vi "nanocal -- nuclear schottky fit V5.vi"() -> ()   [LabVIEW 2020] (continued)
  n20 = Bundle By Name(cluster=T15 {"left"=0.0, "right "=0.0, "center"=0.0, "window"=0.0, "cursors"=[], "relative"=0, "absolute"=0, "fixed vertical offset"=0.0, "vertical offset"=0.0, "skew"=0.0, "default window frac"=0.0, "kind"=enum."symmetric", "skew.left"=0.0, "skew.right"=0.0, "Plot ref"=refnum, "wing order"=enum."forw"} ("cursor bracket: All, data window"), "Plot ref"=w25, "cursors"=i32[] [0, 1, 2], "fixed vertical offset"=0.0, "default window frac"=0.3 ("fixed vertical offset"), "kind"=enum16{"symmetric", "skewed", "fancy"}."symmetric") -> (w28:T15)
  n21 = local write "factors"(cluster{"scaling":dbl, "what":T1}[] [{"scaling"=1.0, "what"=enum."ζ"}, {"scaling"=1.0, "what"=enum."τ1"}, {"scaling"=1.0, "what"=enum."τS"}, {"scaling"=1.0, "what"=enum."τN"}, {"scaling"=1.0, "what"=enum."τC"}, {"scaling"=1.0, "what"=enum."κ0"}]) -> ()
  n22 = control-ref of="cursor window"() -> (w24:refnum<vi>)
  n23 = call "cursor window logic V3.vi"("cursor window action"=cursor_window_action."init", "cursor window in"=w24, "cursor window init"=w28) -> ()  [unwired: 7 in, 2 out]
  n24 = Create User Event(user event datatype=w33) -> (user event=w14:refnum<user-event>)  [unwired: 1 in, 1 out]
  n25 = Bundle(w13, w13) -> (w12:cluster{dbl[], dbl[]})  [unwired: 1 in]
  n26 = Initialize Array(w12, 5 ("dimension size")) -> (→"Plot: goodness vs parameter":cluster{dbl[], dbl[]}[])
  n27 = control-ref of="Plot: sweep window"() -> (w20:refnum<vi>)
  n28 = register-events(w14) -> (reference out=w34:refnum<event-registration>)  [unwired: 2 in, 1 out]
  n29 = Create User Event(user event datatype=w35) -> (user event=w23:refnum<user-event>)  [unwired: 1 in, 1 out]
  n30 = register-events(w23) -> (reference out=w36:refnum<event-registration>)  [unwired: 2 in, 1 out]
  n31 = local write "newton pause"(w16) -> ()
  n32 = control-ref of="Plot:  colors"() -> (w17:refnum<vi>)
  n33 = local write "default selector"(w5) -> ()
  n34 = call "replace cursor - plot ref - V2.vi"("Plot ref in"=w20, "new X"=w19, "new  Y"=w19, "cursor index"=2, "cursor action"=cursor_action."write") -> ()  [unwired: 11 in, 4 out]
  n35 = local write "parameter"(w4) -> ()
  n36 = while "actions" {
    tunnel: w36 -> [w96]
    tunnel: w23 -> [w95]
    tunnel: w14 -> [w93]
    tunnel: w4 -> [w92]
    tunnel: w5 -> [w91]
    stop <- w94 stop-if-true
    n37 = event shown="[0] <action>: User Event" {
      selector: w96 -> [_]
      dyn-events: _ -> [_]
      timeout: _ -> [_]
      tunnel: w95 -> [w101]
      tunnel: [w100] -> w94
      tunnel: w93 -> [w99]
      tunnel: w92 -> [w98]
      tunnel: w91 -> [w97]
      event User Event {
        n38 = event-data() -> ("action"=w102:string)  [unwired: 1 in]
        n39 = case shown="\"action: replot circles\"" w102 {
          tunnel: w101 -> [w114 _ _ w322 w424 w442 w467 _ _ w660 _ w786 _ _ w937 _ w1008 w1100 _ w1157 _ _]
          tunnel: [_ _ _ _ _ _ _ _ _ _ _ _ _ _ _ _ _ _ TRUE _ _ _] -> w100
          tunnel: w99 -> [_ _ _ _ _ _ _ _ _ _ _ _ _ _ _ _ _ _ _ _ _ _]
          tunnel: w98 -> [w105 w174 w202 _ _ _ _ w594 _ _ _ _ _ w833 _ _ w1004 _ _ _ _ _]
          tunnel: w97 -> [_ _ _ _ _ _ _ _ _ _ _ _ _ _ _ _ _ _ _ _ _ _]
          frame "action: new sweep" {
            w117 = T1[] [enum."m1", enum."m2", enum."m3"] items=["ζ", "τ1", "τS", "τN", "τC", "κ0", "m1", "m2", "m3", "T (K)", "B (T)", "θ (deg)", "side (S|R)", "set of (B|T)", "Re(offset)", "Im(offset)"]
            w123 = T1[] [enum."T (K)", enum."B (T)", enum."θ (deg)"] items=["ζ", "τ1", "τS", "τN", "τC", "κ0", "m1", "m2", "m3", "T (K)", "B (T)", "θ (deg)", "side (S|R)", "set of (B|T)", "Re(offset)", "Im(offset)"]
            n40 = local read "τN"() -> (w143:dbl)
            n41 = local read "τC"() -> (w142:dbl)
            n42 = local read "T1"() -> (w145:dbl)
            n43 = local read "κ0"() -> (w141:dbl)
            n44 = local read "τS"() -> (w144:dbl)
            n45 = local read "ζ"() -> (w146:dbl)
            n46 = Generate User Event(user event=w114, event data cluster="action: reset colors" ("event data")) -> ()  [unwired: 2 in, 2 out]
            n47 = Build Array (concatenate)(w105, w117) -> (w116:T1[])
            n48 = Build Array(w146, w145, w144, w143, w142, w141) -> (w129:dbl[])
            n49 = local read "newton parameters"() -> (w110:T2)
            n50 = for {
              shift-right: [w158] -> w106
              shift-left: map{T1, dbl} {} ("Map IN") -> [w159]
              tunnel: w116 -> [w156] mode=indexing
              tunnel: w129 -> [w157] mode=indexing
              tunnel: [w156] -> w118 mode=indexing
              n51 = Insert Into Map(map in=w159, key=w156, value=w157) -> (map out=w158:map{T1, dbl})  [unwired: 2 out]
            }
            n52 = local read "θ (deg)"() -> (w125:dbl)
            n53 = local read "B (T)"() -> (w126:dbl)
            n54 = local read "T (K)"() -> (w127:dbl)
            n55 = call "nanocal -- publish -- freq scan V2.vi"("publisher action"=publisher_action."get") -> ("z out (V)"=w112:cdb[], "data"=w103:T30)  [unwired: 7 in, 2 out]
            n56 = Build Array(w127, w126, w125) -> (w122:dbl[])
            n57 = call "3-lorentzian-heat-response -- V4.vi"("action"=3-lorentzian-heat-response_action."calc m1m2m3", "Map IN"=w106) -> ("Map OUT"=w124:map{T1, dbl})  [unwired: 7 in, 2 out]
            n58 = for {
              shift-right: [w154] -> w121
              shift-left: w124 -> [w155]
              tunnel: w123 -> [w153] mode=indexing
              tunnel: w122 -> [w152] mode=indexing
              n59 = Insert Into Map(map in=w155, key=w153, value=w152) -> (map out=w154:map{T1, dbl})  [unwired: 2 out]
            }
            n60 = control-ref of="Plot: sweep window"() -> (w140:refnum<vi>)
            n61 = call "nanocal -- gradient descent.vi"("data"=w103, "action"=nanocal_--_gradient_descent_--_action."peek", "newton pars"=w110, "parameter keys IN"=w105, "parameter Map IN"=w106) -> ("logarithmic derivatives OUT"=→"logarithmic derivatives":dbl[], "R(ω) out"=w108:cdb[], "goodness OUT"=→"goodness":dbl)  [unwired: 2 in, 2 out]
            n62 = local read "cursor x selector"() -> (w150:map{T1, dbl})
            n63 = local read "X selector"() -> (w149:T1)
            n64 = local read "cursor index map"() -> (w130:map{T1, i32})
            n65 = Complex To Re/Im(x + iy=w112) -> (x=w139:dbl[], y=w138:dbl[])
            n66 = local read "T (K)"() -> (w148:dbl)
            n67 = call "string parse mathematica assosiated array.vi"("action"=mathematica_string_map_action."create string" ("derivative"), "map IN"=w121) -> ("String OUT"=w119:string)  [unwired: 8 in, 1 out]
            n68 = control-ref of="Plot:  colors"() -> (w151:refnum<vi>)
            n69 = local write "String"(w119) -> ()
            n70 = call "replace plot - plot ref - V2.vi"("Plot ref in"=w140, "Array X IN"=w139, "Array Y IN"=w138, "plot index"=enum16{"data R(ω)", "fit R(ω)"}."data R(ω)" ("Plost: sweep window"), "cursor action"=cursor_action."write") -> ("Plot ref out"=w137:refnum<vi>)  [unwired: 11 in, 3 out]
            n71 = Complex To Re/Im(x + iy=w108) -> (x=w135:dbl[], y=w134:dbl[])
            n72 = Look In Map(map=w150, key=w149, default value=w148) -> (value=w147:dbl)  [unwired: 1 out]
            n73 = for {
              tunnel: w147 -> [w167]
              tunnel: w151 -> [w166]
              tunnel: w118 -> [w162] mode=indexing
              tunnel: w130 -> [w164]
              shift-right: [w161] -> _
              shift-left: w124 -> [w161]
              n74 = Look In Map(map=w161, key=w162) -> (value=w160:dbl)  [unwired: 1 in, 1 out]
              n75 = Look In Map(map=w164, key=w162) -> (value=w163:i32)  [unwired: 1 in, 1 out]
              n76 = call "replace cursor - plot ref - V2.vi"("Plot ref in"=w166, "new X"=w167, "new  Y"=w160, "cursor index"=w163, "cursor action"=cursor_action."write") -> ()  [unwired: 11 in, 4 out]
            }
            n77 = call "replace plot - plot ref - V2.vi"("Plot ref in"=w137, "Array X IN"=w135, "Array Y IN"=w134, "plot index"=enum16{"data R(ω)", "fit R(ω)"}."fit R(ω)" ("Plost: sweep window"), "cursor action"=cursor_action."write") -> ()  [unwired: 11 in, 4 out]
          }
          frame "action: replot circles" {
            n78 = local read "τN"() -> (w193:dbl)
            n79 = local read "τC"() -> (w192:dbl)
            n80 = local read "T1"() -> (w195:dbl)
            n81 = local read "κ0"() -> (w191:dbl)
            n82 = local read "τS"() -> (w194:dbl)
            n83 = local read "ζ"() -> (w196:dbl)
            n84 = local read "newton parameters"() -> (w177:T2)
            n85 = Build Array(w196, w195, w194, w193, w192, w191) -> (w171:dbl[])
            n86 = call "nanocal -- publish -- freq scan V2.vi"("publisher action"=publisher_action."get") -> ("z out (V)"=w176:cdb[], "data"=w172:T30)  [unwired: 7 in, 2 out]
            n87 = for {
              shift-right: [w199] -> w173
              shift-left: map{T1, dbl} {} ("Map IN") -> [w200]
              tunnel: w174 -> [w198] mode=indexing
              tunnel: w171 -> [w197] mode=indexing
              n88 = Insert Into Map(map in=w200, key=w198, value=w197) -> (map out=w199:map{T1, dbl})  [unwired: 2 out]
            }
            n89 = call "nanocal -- gradient descent.vi"("data"=w172, "action"=nanocal_--_gradient_descent_--_action."peek", "newton pars"=w177, "parameter keys IN"=w174, "parameter Map IN"=w173) -> ("logarithmic derivatives OUT"=w169:dbl[], "R(ω) out"=w175:cdb[], "goodness OUT"=w170:dbl)  [unwired: 2 in, 2 out]
            n90 = control-ref of="Plot: sweep window"() -> (w188:refnum<vi>)
            n91 = local write "logarithmic derivatives"(w169) -> ()
            n92 = local write "goodness"(w170) -> ()
            n93 = Complex To Re/Im(x + iy=w176) -> (x=w186:dbl[], y=w185:dbl[])
            n94 = call "replace plot - plot ref - V2.vi"("Plot ref in"=w188, "Array X IN"=w186, "Array Y IN"=w185, "plot index"=enum16{"data R(ω)", "fit R(ω)"}."data R(ω)" ("Plost: sweep window"), "cursor action"=cursor_action."write") -> ("Plot ref out"=w187:refnum<vi>)  [unwired: 11 in, 3 out]
            n95 = Complex To Re/Im(x + iy=w175) -> (x=w184:dbl[], y=w183:dbl[])
            n96 = Absolute Value(x=w169) -> (abs(x)=w168:dbl[])
            n97 = local write "log(|dlogG/dlogα|)"(w168) -> ()
            n98 = call "replace plot - plot ref - V2.vi"("Plot ref in"=w187, "Array X IN"=w184, "Array Y IN"=w183, "plot index"=enum16{"data R(ω)", "fit R(ω)"}."fit R(ω)" ("Plost: sweep window"), "cursor action"=cursor_action."write") -> ()  [unwired: 11 in, 4 out]
          }
          frame "action: plot landscape" {
            w214 = array_action."generate log range" ("action")
            n99 = property on="range one" class="Slide (strict)"() -> ("Scale.Range"=w225:T32)  [unwired: 2 in, 2 out]
            n100 = local read "ζ"() -> (w231:dbl)
            n101 = local read "τS"() -> (w229:dbl)
            n102 = local read "τN"() -> (w228:dbl)
            n103 = local read "τC"() -> (w227:dbl)
            n104 = local read "T1"() -> (w230:dbl)
            n105 = local read "κ0"() -> (w226:dbl)
            n106 = property on="range two" class="Slide (strict)"() -> ("Scale.Range"=w224:T32)  [unwired: 2 in, 2 out]
            n107 = Unbundle By Name(w225) -> ("Maximum"=w217:dbl, "Minimum"=w216:dbl)
            n108 = Unbundle By Name(w224) -> ("Maximum"=w219:dbl, "Minimum"=w218:dbl)
            n109 = Build Array(w231, w230, w229, w228, w227, w226) -> (w213:dbl[])
            n110 = local read "cursor index map"() -> (w208:map{T1, i32})
            n111 = call "array -- generate range -- V5.vi"("action"=w214, "ω points"="# points", "ω from"=w216, "ω to"=w217) -> ("ω out"=w215:dbl[])  [unwired: 7 in]
            n112 = call "array -- generate range -- V5.vi"("action"=w214, "ω points"="# points", "ω from"=w218, "ω to"=w219) -> ("ω out"=w220:dbl[])  [unwired: 7 in]
            n113 = local read "color Map"() -> (w209:map{T1, u32})
            n114 = call "nanocal -- publish -- freq scan V2.vi"("publisher action"=publisher_action."get") -> ("data"=w201:T30)  [unwired: 7 in, 3 out]
            n115 = local read "newton parameters"() -> (w203:T2)
            n116 = for {
              shift-right: [w314] -> w221
              shift-left: map{T1, dbl} {} ("Map IN") -> [w315]
              tunnel: w202 -> [w313] mode=indexing
              tunnel: w213 -> [w312] mode=indexing
              n117 = Insert Into Map(map in=w315, key=w313, value=w312) -> (map out=w314:map{T1, dbl})  [unwired: 2 out]
            }
            n118 = Look In Map(map=w209, key="two") -> (value=w211:u32)  [unwired: 1 in, 1 out]
            n119 = Look In Map(map=w209, key="one") -> (value=w210:u32)  [unwired: 1 in, 1 out]
            n120 = Build Array("one", "two") -> (w207:T1[])
            n121 = property on="range one" class="Slide (strict)"("Fill Color"=w210) -> ()  [unwired: 2 in, 2 out]
            n122 = property on="range two" class="Slide (strict)"("Fill Color"=w211) -> ()  [unwired: 2 in, 2 out]
            n123 = case shown="\"1d plots\", Default" "what" {
              tunnel: w221 -> [w239 w279]
              tunnel: "one" -> [_ w278]
              tunnel: w220 -> [_ w277]
              tunnel: w215 -> [w238 w276]
              tunnel: "two" -> [_ w275]
              tunnel: w209 -> [w237 _]
              tunnel: w208 -> [w236 _]
              tunnel: w207 -> [w233 _]
              tunnel: w201 -> [w234 w270]
              tunnel: w203 -> [w232 w268]
              tunnel: w202 -> [_ w269]
              frame "1d plots", Default {
                n124 = control-ref of="Plot: goodness vs parameter"() -> (w235:refnum<vi>)
                n125 = for {
                  tunnel: w239 -> [w246]
                  tunnel: w238 -> [w255]
                  tunnel: w233 -> [w245] mode=indexing
                  tunnel: w237 -> [w252]
                  tunnel: w236 -> [w251]
                  tunnel: w235 -> [w243]
                  tunnel: w234 -> [w242]
                  tunnel: w233 -> [w241]
                  tunnel: w232 -> [w240]
                  n126 = for {
                    tunnel: w255 -> [w259] mode=indexing
                    tunnel: [w260] -> w257 mode=indexing
                    tunnel: [w259] -> w256 mode=indexing
                    tunnel: w246 -> [w266]
                    tunnel: w245 -> [w267]
                    tunnel: w242 -> [w265]
                    tunnel: w241 -> [w262]
                    tunnel: w240 -> [w261]
                    n127 = Insert Into Map(map in=w266, key=w267, value=w259) -> (map out=w264:map{T1, dbl})  [unwired: 2 out]
                    n128 = call "nanocal -- gradient descent.vi"("data"=w265, "action"=nanocal_--_gradient_descent_--_action."peek", "newton pars"=w261, "parameter keys IN"=w262, "parameter Map IN"=w264) -> ("goodness OUT"=w260:dbl)  [unwired: 2 in, 4 out]
                  }
                  n129 = Look In Map(map=w246, key=w245) -> (value=w244:dbl)  [unwired: 1 in, 1 out]
                  n130 = Look In Map(map=w252, key=w245) -> (value=w247:u32)  [unwired: 1 in, 1 out]
                  n131 = Look In Map(map=w251, key=w245) -> (value=w249:i32)  [unwired: 1 in, 1 out]
                  n132 = call "replace plot - plot ref - V2.vi"("Plot ref in"=w243, "Array X IN"=w256, "Array Y IN"=w257, "plot index"=w249, "cursor action"=cursor_action."write") -> ("Plot ref out"=w254:refnum<vi>)  [unwired: 11 in, 3 out]
                  n133 = call "replace cursor - plot ref - V2.vi"("Plot ref in"=w243, "new X"=w244, "cursor index"=w249, "cursor action"=cursor_action."write", "Color Box"=w247, "cursor state"=cursor_sate."colored") -> ()  [unwired: 10 in, 4 out]
                  n134 = call "replace plot - plot ref - V2.vi"("Plot ref in"=w254, "plot index"=w249, "cursor action"=cursor_action."set plot color", "Color Box"=w247) -> ()  [unwired: 12 in, 4 out]
                }
              }
              frame "2d plots " {
                n135 = for {
                  tunnel: w279 -> [w289]
                  tunnel: w278 -> [w288]
                  tunnel: w277 -> [w287] mode=indexing
                  tunnel: w276 -> [w286]
                  tunnel: w275 -> [w285]
                  shift-right: [w283] -> w272
                  shift-left: "{ " -> [w284]
                  tunnel: w270 -> [w282]
                  tunnel: w269 -> [w281]
                  tunnel: w268 -> [w280]
                  n136 = for {
                    tunnel: w286 -> [w297] mode=indexing
                    tunnel: w287 -> [w296]
                    tunnel: w289 -> [w310]
                    tunnel: w288 -> [w311]
                    tunnel: w285 -> [w309]
                    shift-right: [w306] -> w283
                    shift-left: w284 -> [w307]
                    tunnel: w282 -> [w294]
                    tunnel: w281 -> [w291]
                    tunnel: w280 -> [w290]
                    w300 = " ,     "
                    w305 = i16 12 ("precision (6)")
                    n137 = Insert Into Map(map in=w310, key=w311, value=w297) -> (map out=w308:map{T1, dbl})  [unwired: 2 out]
                    n138 = Number To Fractional String(number=w297, precision (6)=w305) -> (F-format string=w304:string)  [unwired: 2 in]
                    n139 = Number To Fractional String(number=w296, precision (6)=w305) -> (F-format string=w303:string)  [unwired: 2 in]
                    n140 = Insert Into Map(map in=w308, key=w309, value=w296) -> (map out=w295:map{T1, dbl})  [unwired: 2 out]
                    n141 = call "nanocal -- gradient descent.vi"("data"=w294, "action"=nanocal_--_gradient_descent_--_action."peek", "newton pars"=w290, "parameter keys IN"=w291, "parameter Map IN"=w295) -> ("goodness OUT"=w292:dbl)  [unwired: 2 in, 4 out]
                    n142 = Number To Fractional String(number=w292, precision (6)=w305) -> (F-format string=w302:string)  [unwired: 2 in]
                    n143 = Concatenate Strings(w307, "{    ", w304, w300, w303, w300, w302, " } , ", "\r") -> (w306:string)
                  }
                }
                n144 = Concatenate Strings(w272, " }   ") -> (→"2dplots":string)
              }
            }
          }
          frame "action: gradient step" {
            w319 = T1[] [enum."ζ", enum."τ1", enum."τS", enum."τN", enum."τC", enum."κ0"] items=["ζ", "τ1", "τS", "τN", "τC", "κ0", "m1", "m2", "m3", "T (K)", "B (T)", "θ (deg)", "side (S|R)", "set of (B|T)", "Re(offset)", "Im(offset)"]
            w323 = FALSE ("newton pause")
            n145 = local write "newton pause"(w323) -> ()
            n146 = call "nanocal -- publish -- freq scan V2.vi"("publisher action"=publisher_action."get") -> ("data"=w316:T30)  [unwired: 7 in, 3 out]
            n147 = Generate User Event(user event=w322, event data cluster="action: new sweep" ("event data")) -> ()  [unwired: 2 in, 2 out]
            n148 = call "nanocal -- gradient descent.vi"("data"=w316, "action"=nanocal_--_gradient_descent_--_action."init") -> ("goodness OUT"=w320:dbl)  [unwired: 5 in, 4 out]
            n149 = for {
              N: "# steps" -> [_]
              tunnel: [TRUE ("newton pause")] -> w324
              tunnel: w323 -> [_]
              tunnel: w320 -> [_]
              tunnel: w319 -> [w332]
              tunnel: map{T1, dbl} {} ("Map IN") -> [w333]
              stop <- w334 stop-if-true
              n150 = local read "ζ"() -> (w369:dbl)
              n151 = local read "T1"() -> (w368:dbl)
              n152 = local read "τS"() -> (w367:dbl)
              n153 = local read "τN"() -> (w366:dbl)
              n154 = local read "τC"() -> (w365:dbl)
              n155 = local read "κ0"() -> (w364:dbl)
              n156 = local read "newton pause"() -> (w334:bool)
              n157 = local read "factors"() -> (w347:cluster{"scaling":dbl, "what":T1}[])
              n158 = local read "newton parameters"() -> (w331:T2)
              n159 = Build Array(w369, w368, w367, w366, w365, w364) -> (w348:dbl[])
              n160 = for {
                shift-right: [w388] -> w346
                shift-left: w333 -> [w389]
                tunnel: w347 -> [w387] mode=indexing
                n161 = Unbundle(w387) -> ("scaling"=w385:dbl, "what"=w386:T1)
                n162 = Insert Into Map(map in=w389, key=w386, value=w385) -> (map out=w388:map{T1, dbl})  [unwired: 2 out]
              }
              n163 = for {
                shift-right: [w392] -> w344
                shift-left: w333 -> [w393]
                tunnel: w332 -> [w390] mode=indexing
                tunnel: w348 -> [w391] mode=indexing
                n164 = Insert Into Map(map in=w393, key=w390, value=w391) -> (map out=w392:map{T1, dbl})  [unwired: 2 out]
              }
              n165 = local read "cursor x selector"() -> (w355:map{T1, dbl})
              n166 = local read "X selector"() -> (w354:T1)
              n167 = call "nanocal -- gradient descent.vi"("# steps"="# osccilation steps", "action"=nanocal_--_gradient_descent_--_action."step", "newton pars"=w331, "parameter keys IN"=w332, "parameter Map IN"=w344, "factors Map IN"=w346) -> ("logarithmic derivatives OUT"=w328:dbl[], "step factors OUT"=w342:map{T1, dbl}, "R(ω) out"=w335:cdb[], "goodness OUT"=w343:dbl, "oscillations"=→"Plot:  goodness oscillations":cluster{"Array":i32[], "Array":dbl[]})  [unwired: 1 in]
              n168 = local read "T (K)"() -> (w353:dbl)
              n169 = local read "cursor index map"() -> (w351:map{T1, i32})
              n170 = call "3-lorentzian-heat-response -- V4.vi"("action"=3-lorentzian-heat-response_action."calc m1m2m3", "Map IN"=w344) -> ("Map OUT"=w350:map{T1, dbl})  [unwired: 7 in, 2 out]
              n171 = control-ref of="Plot:  colors"() -> (w356:refnum<vi>)
              n172 = for {
                tunnel: w332 -> [w384] mode=indexing
                shift-right: [w383] -> _
                shift-left: w342 -> [w383]
                tunnel: [w382] -> w341 mode=indexing
                n173 = Look In Map(map=w383, key=w384) -> (value=w382:dbl)  [unwired: 1 in, 1 out]
              }
              n174 = Look In Map(map=w355, key=w354, default value=w353) -> (value=w352:dbl)  [unwired: 1 out]
              n175 = for {
                tunnel: w352 -> [w401]
                tunnel: w356 -> [w400]
                tunnel: w332 -> [w396] mode=indexing
                tunnel: w351 -> [w398]
                shift-right: [w395] -> _
                shift-left: w350 -> [w395]
                n176 = Look In Map(map=w395, key=w396) -> (value=w394:dbl)  [unwired: 1 in, 1 out]
                n177 = Look In Map(map=w398, key=w396) -> (value=w397:i32)  [unwired: 1 in, 1 out]
                n178 = call "replace cursor - plot ref - V2.vi"("Plot ref in"=w400, "new X"=w401, "new  Y"=w394, "cursor index"=w397, "cursor action"=cursor_action."write") -> ()  [unwired: 11 in, 4 out]
              }
              n179 = Index Array(array=w341, index #1=0 ("index"), index #2=1 ("index"), index #3=2 ("index"), index #4=3 ("index"), index #5=4 ("index"), index #6=5 ("index")) -> (element #1=w376:dbl, element #2=w375:dbl, element #3=w374:dbl, element #4=w373:dbl, element #5=w372:dbl, element #6=w370:dbl)
              n180 = Multiply(x=w376, y=w369) -> (x*y=w381:dbl)
              n181 = local write "goodness"(w343) -> ()
              n182 = local write "logarithmic derivatives"(w328) -> ()
              n183 = Multiply(x=w375, y=w368) -> (x*y=w380:dbl)
              n184 = Absolute Value(x=w328) -> (abs(x)=→"log(|dlogG/dlogα|)":dbl[])
              n185 = Multiply(x=w374, y=w367) -> (x*y=w379:dbl)
              n186 = Complex To Re/Im(x + iy=w335) -> (x=w359:dbl[], y=w358:dbl[])
              n187 = Multiply(x=w373, y=w366) -> (x*y=w378:dbl)
              n188 = control-ref of="Plot: sweep window"() -> (w361:refnum<vi>)
              n189 = Multiply(x=w372, y=w365) -> (x*y=w377:dbl)
              n190 = Multiply(x=w370, y=w364) -> (x*y=w371:dbl)
              n191 = call "replace plot - plot ref - V2.vi"("Plot ref in"=w361, "Array X IN"=w359, "Array Y IN"=w358, "plot index"=enum16{"data R(ω)", "fit R(ω)"}."fit R(ω)" ("Plost: sweep window"), "cursor action"=cursor_action."write") -> ()  [unwired: 11 in, 4 out]
              n192 = local write "ζ"(w381) -> ()
              n193 = local write "T1"(w380) -> ()
              n194 = local write "τS"(w379) -> ()
              n195 = local write "τN"(w378) -> ()
              n196 = local write "τC"(w377) -> ()
              n197 = local write "κ0"(w371) -> ()
            }
            n198 = local write "newton pause"(w324) -> ()
          }
          frame "action: uco" {
            (unwired) 3-lorentzian-parameters."κ0" ("Plost: sweep window")
            n199 = local read "T1"() -> (w416:dbl)
            n200 = local read "τN"() -> (w414:dbl)
            n201 = local read "τC"() -> (w413:dbl)
            n202 = local read "τS"() -> (w415:dbl)
            n203 = local read "κ0"() -> (w412:dbl)
            n204 = local read "ζ"() -> (w417:dbl)
            n205 = Generate User Event(user event=w424, event data cluster="action: new sweep" ("event data")) -> ()  [unwired: 2 in, 2 out]
            n206 = call "3-lorentzian-parameters - manage.vi"("ζ"=w417, "T1"=w416, "τS"=w415, "τN"=w414, "τC"=w413, "κ0"=w412, "parameters"=3-lorentzian-parameters_--_action."to array") -> ("parameter array OUT"=w410:dbl[])  [unwired: 6 in, 6 out]
            n207 = Natural Logarithm(1:w410) -> (0:w422:dbl[])
            n208 = vi-ref "nanocal -- nuclear schottky goodness -- for UCO -- V3.vi"() -> (w423:refnum<vi>)
            n209 = call-poly <vilib>:"Unconstrained Optimization.vi"("function data"=T23 variant, "objective function"=w423, "start"=w422) -> ("f(minimum)"=w420:dbl, "minimum"=w421:dbl[])  [unwired: 5 in, 2 out]
            n210 = Exponential(1:w420) -> (0:w419:dbl)
            n211 = Exponential(1:w421) -> (0:w409:dbl[])
            n212 = call "3-lorentzian-parameters - manage.vi"("parameter array"=w409, "parameters"=3-lorentzian-parameters_--_action."to parameters") -> ("ζ OUT"=w408:dbl, "T1 OUT"=w407:dbl, "τS  OUT"=w406:dbl, "τN  OUT"=w405:dbl, "τC  OUT"=w404:dbl, "κ0  OUT"=w403:dbl)  [unwired: 11 in, 1 out]
            n213 = local write "goodness"(w419) -> ()
            n214 = local write "T1"(w407) -> ()
            n215 = local write "τN"(w405) -> ()
            n216 = local write "τC"(w404) -> ()
            n217 = local write "τS"(w406) -> ()
            n218 = local write "κ0"(w403) -> ()
            n219 = local write "ζ"(w408) -> ()
          }
          frame "action: parse string" {
            n220 = local read "String"() -> (w444:string)
            n221 = call "string parse mathematica assosiated array.vi"("action"=mathematica_string_map_action."parse string" ("derivative"), "String in"=w444) -> ("Map OUT"=w438:map{T1, dbl})  [unwired: 8 in, 1 out]
            n222 = Generate User Event "action User Event"(user event=w442, event data cluster="action: update state of selectors" ("event data")) -> (user event out=w426:refnum<user-event>)  [unwired: 2 in, 1 out]
            n223 = Look In Map(map=w438, key=3-lorentzian-parameters."ζ" ("Plost: sweep window")) -> (value=w433:dbl)  [unwired: 1 in, 1 out]
            n224 = Look In Map(map=w438, key=3-lorentzian-parameters."τ1" ("Plost: sweep window")) -> (value=w432:dbl)  [unwired: 1 in, 1 out]
            n225 = Look In Map(map=w438, key=3-lorentzian-parameters."τS" ("Plost: sweep window")) -> (value=w431:dbl)  [unwired: 1 in, 1 out]
            n226 = Look In Map(map=w438, key=3-lorentzian-parameters."τN" ("Plost: sweep window")) -> (value=w430:dbl)  [unwired: 1 in, 1 out]
            n227 = Look In Map(map=w438, key=3-lorentzian-parameters."τC" ("Plost: sweep window")) -> (value=w429:dbl)  [unwired: 1 in, 1 out]
            n228 = Look In Map(map=w438, key=3-lorentzian-parameters."κ0" ("Plost: sweep window")) -> (value=w428:dbl)  [unwired: 1 in, 1 out]
            n229 = local write "ζ"(w433) -> ()
            n230 = local write "τS"(w431) -> ()
            n231 = local write "τN"(w430) -> ()
            n232 = local write "τC"(w429) -> ()
            n233 = local write "T1"(w432) -> ()
            n234 = local write "κ0"(w428) -> ()
            n235 = Generate User Event "action User Event"(user event=w426, event data cluster="action: replot colors" ("event data")) -> ()  [unwired: 2 in, 2 out]
          }
          frame "action: read mathematica string" {
            w453 = map{string, path} {}  # Size: 0
            w469 = map{T1, dbl} {}  # Size: 0
            w466 = set{dbl} {}  # Size: 0
            w470 = map{string, map{T1, dbl}} {}  # Size: 0
            w459 = map{string, string} {}  # Size: 0
            n236 = local read "file pattern"() -> (w456:string)
            n237 = local read "data file parameters map"() -> (w462:map{T1, T9})
            n238 = local read "folder"() -> (w457:path)
            n239 = local read "side map to NUM"() -> (w460:map{T8, i32})
            n240 = call <vilib>:"Recursive File List.vi"("pattern"=w456, "Continue Recursing on Error? (F)"=TRUE, "Folder Path"=w457) -> ("All Files in Dir"=w454:path[])  [unwired: 4 in, 4 out]
            n241 = call "string parse mathematica list assosiated array -- V2.vi"("action"=3-lorentzian-heat-response_action."parse string" ("derivative"), "string IN"="string IN") -> ("Map OUT"=w471:map{string, map{T1, dbl}})  [unwired: 8 in, 1 out]
            n242 = local read "side map to STR"() -> (w461:map{T8, string})
            n243 = Generate User Event(user event=w467, event data cluster="action: update enums" ("event data")) -> ()  [unwired: 2 in, 2 out]
            n244 = for {
              tunnel: w454 -> [w479] mode=indexing
              shift-right: [w493] -> w463
              shift-left: w471 -> [w503]
              shift-right: [w490] -> w465
              shift-left: w459 -> [w502]
              shift-right: [w489] -> w464
              shift-left: w470 -> [w498]
              shift-right: [w500] -> w448
              shift-left: w466 -> [w492]
              shift-right: [w491] -> w447
              shift-left: w466 -> [w501]
              tunnel: w469 -> [w496]
              shift-right: [w486] -> w446
              shift-left: w466 -> [w499]
              shift-right: [w488] -> w449
              shift-left: w466 -> [w497]
              tunnel: w462 -> [w495]
              shift-right: [w487] -> w451
              shift-left: w466 -> [w494]
              tunnel: w460 -> [w484]
              tunnel: w461 -> [w483]
              shift-right: [w480] -> w458
              shift-left: w453 -> [w481]
              w482 = T8[] [enum."sam", enum."ref"] items=["sam", "ref"]
              n245 = Strip Path(path=w479) -> (name=w478:string)  [unwired: 1 out]
              n246 = call "filename-manage.vi"("filename-action"=filename-action."getIDStock", "file name IN"=w478) -> ("string OUT"=w485:string)  [unwired: 7 in, 2 out]
              n247 = for {
                tunnel: w495 -> [w529]
                tunnel: w478 -> [w506]
                tunnel: w485 -> [w518]
                shift-right: [w527] -> w493
                shift-left: w503 -> [w538]
                shift-right: [w533] -> w500
                shift-left: w492 -> [w526]
                shift-right: [w525] -> w491
                shift-left: w501 -> [w534]
                shift-right: [w519] -> w486
                shift-left: w499 -> [w532]
                shift-right: [w520] -> w488
                shift-left: w497 -> [w530]
                shift-right: [w521] -> w487
                shift-left: w494 -> [w528]
                shift-right: [w522] -> w489
                shift-left: w498 -> [w531]
                shift-right: [w523] -> w490
                shift-left: w502 -> [w537]
                tunnel: w484 -> [w511]
                tunnel: w496 -> [w516]
                tunnel: w483 -> [w513]
                tunnel: w482 -> [w510] mode=indexing
                shift-right: [w507] -> w480
                shift-left: w481 -> [w508]
                tunnel: w479 -> [w505]
                # "internal key"
                n248 = Look In Map(map=w513, key=w510) -> (value=w512:string)  [unwired: 1 in, 1 out]
                n249 = Look In Map(map=w511, key=w510) -> (value=w509:i32)  [unwired: 1 in, 1 out]
                n250 = Concatenate Strings(w518, w512) -> (w517:string)
                n251 = Insert Into Map(map in=w516, key=3-lorentzian-parameters."side (S|R)", value=w509) -> (map out=w515:map{T1, dbl})  [unwired: 2 out]
                n252 = for {
                  shift-right: [w544] -> w524
                  shift-left: w515 -> [w545]
                  tunnel: w529 -> [w543] mode=indexing
                  tunnel: w506 -> [w541]
                  n253 = Unbundle(w543) -> ("key"=w542:T1, "filename-action"=w540:T9)
                  n254 = call "filename-manage.vi"("filename-action"=w540, "file name IN"=w541) -> ("number OUT"=w539:dbl)  [unwired: 7 in, 2 out]
                  n255 = Insert Into Map(map in=w545, key=w542, value=w539) -> (map out=w544:map{T1, dbl})  [unwired: 2 out]
                }
                n256 = in-place {
                  in-place-border: [w587] -> w536
                  in-place-border: w524 -> [w586]
                  n257 = in-place-map #1(w538, w517) -> (w585:map{T1, dbl}, w587:bool)  [unwired: 1 in]
                  n258 = for {
                    tunnel: w586 -> [w593] mode=indexing
                    shift-right: [w591] -> w584
                    shift-left: w585 -> [w592]
                    n259 = Unbundle(w593) -> ("key"=w590:T1, "number OUT"=w589:dbl)
                    n260 = Insert Into Map(map in=w592, key=w590, value=w589) -> (map out=w591:map{T1, dbl})  [unwired: 2 out]
                  }
                  n261 = in-place-map #1(w584, LVMapReplaceAction."Modify Entry only if found" ("action")) -> (w527:map{string, map{T1, dbl}})  [unwired: 2 out]
                }
                n262 = Not(x=w536) -> (.not. x?=w535:bool)
                n263 = case shown="True" w535 {
                  tunnel: w537 -> [w553 w583]
                  tunnel: [w553 w582] -> w523
                  tunnel: w506 -> [_ w581]
                  tunnel: w517 -> [_ w555]
                  tunnel: w534 -> [w551 w580]
                  tunnel: [w551 w579] -> w525
                  tunnel: w526 -> [w552 w578]
                  tunnel: [w552 w577] -> w533
                  tunnel: [w549 w576] -> w519
                  tunnel: w532 -> [w549 w575]
                  tunnel: w524 -> [_ w560]
                  tunnel: w531 -> [w550 w574]
                  tunnel: [w550 w573] -> w522
                  tunnel: [w548 w572] -> w520
                  tunnel: w530 -> [w548 w571]
                  tunnel: [w547 w562] -> w521
                  tunnel: w528 -> [w547 w561]
                  tunnel: w508 -> [w546 w557]
                  tunnel: [w546 w556] -> w507
                  tunnel: w505 -> [_ w554]
                  frame False {
                  }
                  frame True {
                    n264 = Look In Map(map=w560, key=3-lorentzian-parameters."set of (B|T)") -> (value=w563:dbl)  [unwired: 1 in, 1 out]
                    n265 = Look In Map(map=w560, key=3-lorentzian-parameters."side (S|R)") -> (value=w569:dbl)  [unwired: 1 in, 1 out]
                    n266 = Look In Map(map=w560, key=3-lorentzian-parameters."T (K)") -> (value=w567:dbl)  [unwired: 1 in, 1 out]
                    n267 = Look In Map(map=w560, key=3-lorentzian-parameters."B (T)") -> (value=w559:dbl)  [unwired: 1 in, 1 out]
                    n268 = Look In Map(map=w560, key=3-lorentzian-parameters."θ (deg)") -> (value=w558:dbl)  [unwired: 1 in, 1 out]
                    n269 = Insert Into Set(10:w563, 11:w561) -> (3:w562:set{dbl})  [unwired: 1 out]
                    n270 = Insert Into Set(10:w569, 11:w571) -> (3:w572:set{dbl})  [unwired: 1 out]
                    n271 = Insert Into Set(10:w567, 11:w575) -> (3:w576:set{dbl})  [unwired: 1 out]
                    n272 = Insert Into Set(10:w559, 11:w580) -> (3:w579:set{dbl})  [unwired: 1 out]
                    n273 = Insert Into Set(10:w558, 11:w578) -> (3:w577:set{dbl})  [unwired: 1 out]
                    n274 = Insert Into Map(map in=w574, key=w555, value=w560) -> (map out=w573:map{string, map{T1, dbl}})  [unwired: 2 out]
                    n275 = Insert Into Map(map in=w583, key=w555, value=w581) -> (map out=w582:map{string, string})  [unwired: 2 out]
                    n276 = Insert Into Map(map in=w557, key=w555, value=w554) -> (map out=w556:map{string, path})  [unwired: 2 out]
                  }
                }
              }
            }
            "all short filenames" <- w465
            "temps&degs" <- w464
            "all full filenames" <- w458
            n277 = local write "mathematica thing"(w463) -> ()
            n278 = local read "selector"() -> (w452:T12)
            n279 = in-place {
              in-place-border: w451 -> [w477]
              in-place-border: w449 -> [w476]
              in-place-border: w448 -> [w473]
              in-place-border: w447 -> [w474]
              in-place-border: w446 -> [w475]
              n280 = in-place-cluster #2(w452) -> ()  [unwired: 5 out]
              n281 = in-place-cluster #2("lookup.all set of"=w477, "lookup.all sides"=w476, "lookup.all T's"=w475, "lookup.all B's"=w474, "lookup.all θ's"=w473) -> (w450:T12)
            }
            n282 = local write "selector"(w450) -> ()
          }
          frame "action: update default values" {
            w598 = map{T1, cluster{"ζ":dbl, "ζ":dbl}[]} {}  # Size: 0
            (unwired) map{string, map{T1, dbl}} {} ("Map OUT")
            w596 = map{T1, dbl[]} {}  # Size: 0
            n283 = call "string parse mathematica list assosiated array -- V2.vi"("action"=3-lorentzian-heat-response_action."parse string" ("derivative"), "string IN"="default values string") -> ("Map OUT"=w599:map{string, map{T1, dbl}})  [unwired: 8 in, 1 out]
            n284 = for {
              tunnel: w599 -> [w625] mode=indexing
              tunnel: w594 -> [w624]
              shift-right: [w622] -> w597
              shift-left: w598 -> [w621]
              n285 = Unbundle(w625) -> ("Map"=w623:map{T1, dbl})  [unwired: 1 out]
              n286 = for {
                tunnel: w624 -> [w633] mode=indexing
                tunnel: w623 -> [w632]
                shift-right: [w627] -> w622
                shift-left: w621 -> [w626]
                # "parameter"
                # "temperastures"
                n287 = Look In Map(map=w632, key=w633) -> (value=w629:dbl)  [unwired: 1 in, 1 out]
                n288 = Look In Map(map=w626, key=w633) -> (value=w635:cluster{"ζ":dbl, "ζ":dbl}[])  [unwired: 1 in, 1 out]
                n289 = Look In Map(map=w632, key=3-lorentzian-parameters."T (K)" ("Plost: sweep window")) -> (value=w630:dbl)  [unwired: 1 in, 1 out]
                n290 = Bundle("ζ"=w630, "ζ"=w629) -> (w628:cluster{"ζ":dbl, "ζ":dbl})  [unwired: 1 in]
                n291 = Build Array (concatenate)(w635, w628) -> (w634:cluster{"ζ":dbl, "ζ":dbl}[])
                n292 = Insert Into Map(map in=w626, key=w633, value=w634) -> (map out=w627:map{T1, cluster{"ζ":dbl, "ζ":dbl}[]})  [unwired: 2 out]
              }
            }
            n293 = for {
              tunnel: w597 -> [w614] mode=indexing
              shift-right: [w611] -> w595
              shift-left: w596 -> [w610]
              # "sorted temperastures"
              # "parameter"
              # "temperastures"
              n294 = Unbundle(w614) -> ("Plost: sweep window"=w608:T1, w613:cluster{"ζ":dbl, "ζ":dbl}[])
              n295 = for {
                tunnel: w613 -> [w620] mode=indexing
                tunnel: [w619] -> w612 mode=indexing
                tunnel: [w618] -> w605 mode=indexing
                n296 = Unbundle(w620) -> ("ζ"=w619:dbl, "ζ"=w618:dbl)
              }
              n297 = call "array - sorted inexes.vi"("x"=w612) -> ("index array"=w604:i32[], "sorted array"=w606:dbl[])  [unwired: 9 in]
              n298 = Insert Into Map(map in=w610, key=3-lorentzian-parameters."T (K)", value=w606) -> (map out=w609:map{T1, dbl[]})  [unwired: 2 out]
              n299 = for {
                tunnel: w605 -> [w617]
                tunnel: w604 -> [w616] mode=indexing
                tunnel: [w615] -> w603 mode=indexing
                n300 = Index Array(array=w617, index=w616) -> (element=w615:dbl)
              }
              n301 = Insert Into Map(map in=w609, key=w608, value=w603) -> (map out=w611:map{T1, dbl[]})  [unwired: 2 out]
            }
            n302 = disable-structure shown="Disabled" {
              frame Disabled {
                # "2 3 4 0 1"
                # "2 3 4 5 6"
                # "5 6 2 3 4"
                n303 = call "array - sorted inexes.vi"() -> ()  [unwired: 10 in, 2 out]
              }
              frame Enabled {
              }
            }
            n304 = call "nanocal -- defaut parameter manager -- V1.vi"("action"=nanocal_--_defaut_parameter_manager_action--_V1."update", "internal map"=w595) -> ()  [unwired: 9 in, 1 out]
          }
          frame "action: empty string from filelist" {
            n305 = local read "file pattern"() -> (w637:string)
            n306 = local read "folder"() -> (w638:path)
            n307 = call <vilib>:"Recursive File List.vi"("pattern"=w637, "Continue Recursing on Error? (F)"=TRUE, "Folder Path"=w638) -> ("All Files in Dir"=w636:path[])  [unwired: 4 in, 4 out]
            n308 = for {
              tunnel: [w643] -> w640 mode=concatenating
              tunnel: w636 -> [w648] mode=indexing
              w646 = T8[] [enum."ref", enum."sam"] items=["sam", "ref"]
              n309 = Strip Path(path=w648) -> (name=w647:string)  [unwired: 1 out]
              n310 = local read "side map to STR"() -> (w645:map{T8, string})
              n311 = call "filename-manage.vi"("filename-action"=filename-action."getIDStock", "file name IN"=w647) -> ("string OUT"=w644:string)  [unwired: 7 in, 2 out]
              n312 = for {
                tunnel: w646 -> [w653] mode=indexing
                tunnel: w645 -> [w654]
                tunnel: w644 -> [w652]
                tunnel: [w650] -> w643 mode=indexing
                n313 = Look In Map(map=w654, key=w653) -> (value=w651:string)  [unwired: 1 in, 1 out]
                n314 = Concatenate Strings(w652, w651) -> (w650:string)
              }
            }
            n315 = call "string parse mathematica list assosiated array -- V2.vi"("action"=3-lorentzian-heat-response_action."create emty string" ("derivative"), "array of IDs"=w640) -> ("string out"=w641:string)  [unwired: 8 in, 1 out]
            n316 = local write "string OUT"(w641) -> ()
          }
          frame "action: update enums" {
            w658 = map{string, string} {}  # Size: 0
            w664 = map{i32, string} {}  # Size: 0
            # "gives a key"
            n317 = local read "selector"() -> (w656:T12)
            n318 = Generate User Event(user event=w660, event data cluster="action: update state of selectors" ("event data")) -> ()  [unwired: 2 in, 2 out]
            n319 = local read "all short filenames"() -> (w659:map{string, string})
            n320 = in-place {
              w681 = map{i32, dbl} {}  # Size: 0
              w687 = map{i32, dbl} {}  # Size: 0
              w688 = map{i32, dbl} {}  # Size: 0
              w690 = map{i32, dbl} {}  # Size: 0
              w689 = map{i32, dbl} {}  # Size: 0
              n321 = in-place-cluster #3(w656) -> ("lookup.all set of"=w675:set{dbl}, "lookup.all sides"=w674:set{dbl}, "lookup.all T's"=w673:set{dbl}, "lookup.all θ's"=w672:set{dbl}, "lookup.all B's"=w671:set{dbl})  [unwired: 5 out]
              n322 = for {
                shift-right: [w694] -> w680
                shift-left: w681 -> [w695]
                tunnel: [w692] -> w682 mode=indexing
                tunnel: w675 -> [w691] mode=indexing
                i -> [w693]
                n323 = Number To Decimal String(number=w691) -> (decimal integer string=w692:string)  [unwired: 1 in]
                n324 = Insert Into Map(map in=w695, key=w693, value=w691) -> (map out=w694:map{i32, dbl})  [unwired: 2 out]
              }
              n325 = for {
                shift-right: [w705] -> w677
                shift-left: w688 -> [w706]
                tunnel: [w703] -> w684 mode=indexing
                tunnel: w673 -> [w702] mode=indexing
                i -> [w704]
                n326 = Number To Fractional String(number=w702, precision (6)=i16 3) -> (F-format string=w703:string)  [unwired: 2 in]
                n327 = Insert Into Map(map in=w706, key=w704, value=w702) -> (map out=w705:map{i32, dbl})  [unwired: 2 out]
              }
              n328 = property on="set (1T|2B)" class="Ring (strict)"("Strings []"=w682) -> ()  [unwired: 2 in, 2 out]
              n329 = property on="T (K)" class="Ring (strict)"("Strings []"=w684) -> ()  [unwired: 2 in, 2 out]
              n330 = for {
                shift-right: [w699] -> w679
                shift-left: w687 -> [w700]
                tunnel: [w697] -> w683 mode=indexing
                tunnel: w674 -> [w696] mode=indexing
                i -> [w698]
                n331 = Number To Decimal String(number=w696) -> (decimal integer string=w697:string)  [unwired: 1 in]
                n332 = Insert Into Map(map in=w700, key=w698, value=w696) -> (map out=w699:map{i32, dbl})  [unwired: 2 out]
              }
              n333 = property on="side (8S|4R)" class="Ring (strict)"("Strings []"=w683) -> ()  [unwired: 2 in, 2 out]
              n334 = for {
                shift-right: [w717] -> w676
                shift-left: w689 -> [w718]
                tunnel: [w715] -> w685 mode=indexing
                tunnel: w672 -> [w714] mode=indexing
                i -> [w716]
                n335 = Number To Fractional String(number=w714, precision (6)=i16 3) -> (F-format string=w715:string)  [unwired: 2 in]
                n336 = Insert Into Map(map in=w718, key=w716, value=w714) -> (map out=w717:map{i32, dbl})  [unwired: 2 out]
              }
              n337 = for {
                shift-right: [w711] -> w678
                shift-left: w690 -> [w712]
                tunnel: [w709] -> w686 mode=indexing
                tunnel: w671 -> [w708] mode=indexing
                i -> [w710]
                n338 = Number To Fractional String(number=w708, precision (6)=i16 3) -> (F-format string=w709:string)  [unwired: 2 in]
                n339 = Insert Into Map(map in=w712, key=w710, value=w708) -> (map out=w711:map{i32, dbl})  [unwired: 2 out]
              }
              n340 = property on="θ (deg)" class="Ring (strict)"("Strings []"=w685) -> ()  [unwired: 2 in, 2 out]
              n341 = property on="B (T)" class="Ring (strict)"("Strings []"=w686) -> ()  [unwired: 2 in, 2 out]
              n342 = in-place-cluster #3("lookup.all set of"=w675, "lookup.all sides"=w674, "lookup.all T's"=w673, "lookup.all θ's"=w672, "lookup.all B's"=w671, "lookup.set of lookup"=w680, "lookup.side lookup"=w679, "lookup.T lookup"=w677, "lookup.B lookup"=w678, "lookup.θ lookup"=w676) -> (w655:T12)
            }
            n343 = for {
              tunnel: w659 -> [w723] mode=indexing
              shift-right: [w721] -> w657
              shift-left: w658 -> [w722]
              n344 = Unbundle(w723) -> ("event data"=w719:string, "file pattern"=w720:string)
              n345 = Insert Into Map(map in=w722, key=w720, value=w719) -> (map out=w721:map{string, string})  [unwired: 2 out]
            }
            n346 = local read "temps&degs"() -> (w663:map{string, map{T1, dbl}})
            n347 = local read "X selector"() -> (w662:T1)
            n348 = for {
              tunnel: [w732] -> w667 mode=indexing
              tunnel: [w736] -> w665 mode=indexing
              tunnel: [w733] -> w669 mode=indexing
              tunnel: w662 -> [w737]
              tunnel: w657 -> [w735] mode=indexing
              tunnel: w663 -> [w734]
              n349 = Unbundle(w735) -> (w732:string, w733:string)
              n350 = Look In Map(map=w734, key=w733) -> (value=w738:map{T1, dbl})  [unwired: 1 in, 1 out]
              n351 = Look In Map(map=w738, key=w737) -> (value=w736:dbl)  [unwired: 1 in, 1 out]
            }
            n352 = call "array - sorted inexes.vi"("x"=w665) -> ("index array"=w666:i32[])  [unwired: 9 in, 1 out]
            n353 = for {
              tunnel: w666 -> [w728] mode=indexing
              tunnel: w667 -> [w731]
              tunnel: [w730] -> w668 mode=indexing
              tunnel: w669 -> [w729]
              shift-right: [w724] -> w670
              shift-left: w664 -> [w727]
              i -> [w726]
              n354 = Index Array(array=w731, index=w728) -> (element=w730:string)
              n355 = Index Array(array=w729, index=w728) -> (element=w725:string)
              n356 = Insert Into Map(map in=w727, key=w726, value=w725) -> (map out=w724:map{i32, string})  [unwired: 2 out]
            }
            "filesnames lookup" <- w670
            n357 = property on="filenames" class="Ring (strict)"("Strings []"=w668) -> ()  [unwired: 2 in, 2 out]
            n358 = local write "selector"(w655) -> ()
          }
          frame "action: update constrained file selector" {
            w745 = map{i32, string} {}  # Size: 0
            n359 = local read "state of all selectors"() -> (w741:map{T1, map{bool, dbl}})
            n360 = local read "all short filenames"() -> (w742:map{string, string})
            n361 = local read "temps&degs"() -> (w743:map{string, map{T1, dbl}})
            n362 = for {
              tunnel: w742 -> [w755] mode=indexing
              tunnel: [w755] -> w744 mode=indexing if=w752
              shift-right: [w754] -> w740
              shift-left: w743 -> [w754]
              tunnel: w741 -> [w751]
              n363 = for {
                tunnel: [w767] -> w753 mode=indexing
                shift-right: [w762] -> _
                shift-left: w755 -> [w762]
                shift-right: [w761] -> _
                shift-left: w754 -> [w761]
                tunnel: w751 -> [w760] mode=indexing
                n364 = Unbundle(w762) -> ("event data"=w766:string)  [unwired: 1 out]
                n365 = Unbundle(w760) -> ("Plost: sweep window"=w759:T1, "map"=w758:map{bool, dbl})
                n366 = for {
                  tunnel: w758 -> [w770] mode=indexing
                  tunnel: [w769] -> w756
                  tunnel: [w768] -> w757
                  n367 = Unbundle(w770) -> ("ignore side !"=w769:bool, "number OUT"=w768:dbl)
                }
                n368 = Look In Map(map=w761, key=w766) -> (value=w765:map{T1, dbl})  [unwired: 1 in, 1 out]
                n369 = Look In Map(map=w765, key=w759) -> (value=w764:dbl)  [unwired: 1 in, 1 out]
                n370 = Equal?(x=w764, y=w757) -> (x = y?=w763:bool)
